vi "Remote Reset.vi"() -> ()   [LabVIEW 2011]
doc: "Resets a remote RT target.\n\n\nVersion 1.0 - 02/13/2013\n\nPhaeron, Inc.\nwww.phaeron.com\ninfo@phaeron.com"
uses:
  <vilib>/real-time/NI_Real-Time Libraries.lvlib
  <vilib>/real-time/rtutility.llb/RT Restart Target (IP).vi
panel:
  in  "RT Target Location":string="192.168.x.x"
  out "error out":errorcluster
  in  "Stop Button":bool
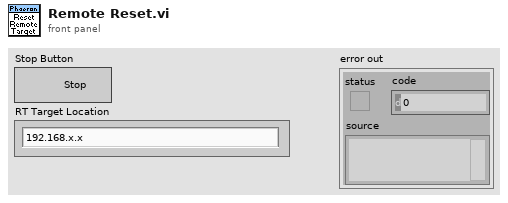
[diagram p1: front panel]
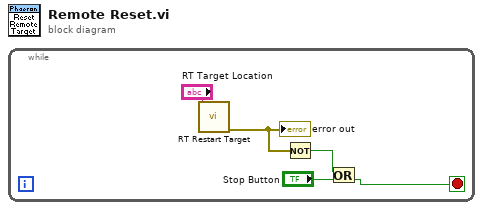
[diagram p0: block diagram]
diagram:
  n1 = while {
    stop <- w3 stop-if-true
    n2 = call-poly <vilib>:"RT Restart Target.vi"("target address"="RT Target Location") -> ("error out"=w2:errorcluster)  [unwired: 8 in, 2 out]
    "error out" <- w2
    n3 = Not(x=w2) -> (.not. x?=w1:bool)
    n4 = Or(x=w1, y="Stop Button") -> (x .or. y?=w3:bool)
  }
